vi "SaveWaveform.vi"(10 "Waveform Chart":waveform(dbl)(graph), 11 "file path (dialog if empty)":path=path "D:/Data/Mai/test target/waveformtest") -> (0 "error out":errorcluster)   [LabVIEW 2018, in "RW_Protocols.lvlib"]
uses:
  RW_Protocols.lvlib
  <vilib>/Waveform/WDTFileIO.llb/Export Waveforms To Spreadsheet File (1D).vi
panel:
  out "History Data":waveform(dbl)[](array[waveform])
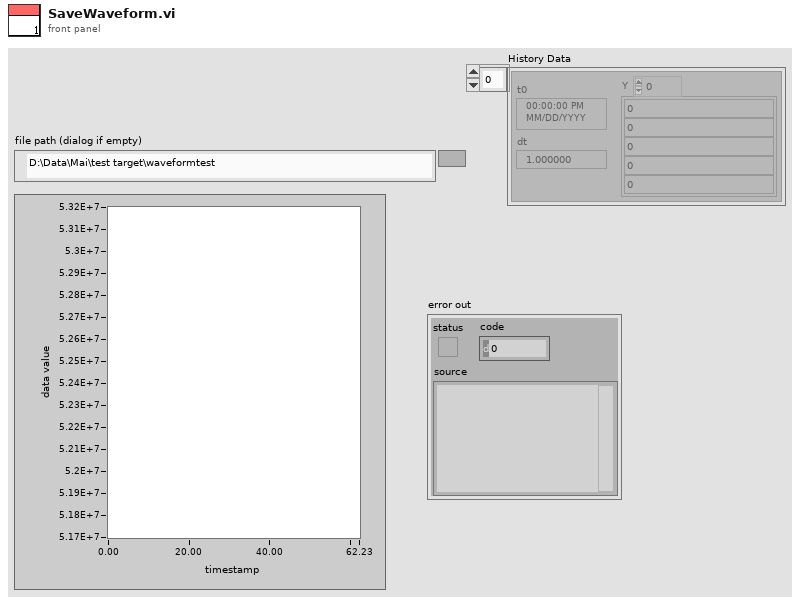
[diagram p1: front panel]
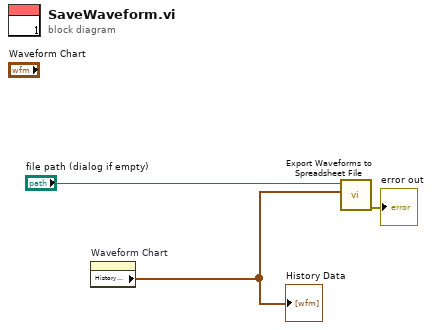
[diagram p0: block diagram]
diagram:
  n1 = property on="Waveform Chart" class="WFChart (strict)"() -> ("History Data"=w1:waveform(dbl)[])  [unwired: 2 in, 2 out]
  "History Data" <- w1
  n2 = call-poly <vilib>:"Export Waveforms to Spreadsheet File.vi"("waveforms"=w1, "file path (dialog if empty)"="file path (dialog if empty)") -> ("error out"=→"error out":errorcluster)  [unwired: 8 in, 1 out]
